vi "Exercise 1.vi"() -> ()   [LabVIEW 2017]
panel:
  out "Result":dbl
  in  "Operand 2":dbl
  in  "Operand 1":dbl
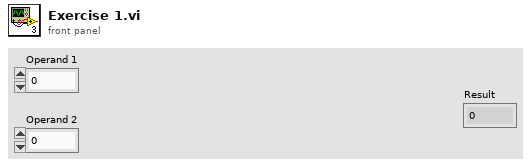
[diagram p1: front panel]
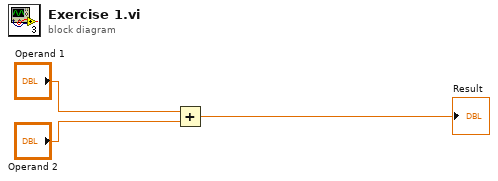
[diagram p0: block diagram]
diagram:
  n1 = Add(x="Operand 1", y="Operand 2") -> (x+y=→"Result":dbl)
